vi "LED 2V2.vi"(0 "Digital IO in":T2, 5 "LED Red":bool, 9 "LED Green":bool, 11 "error in (no error)":errorcluster, 12 "LED Red 2":bool, 13 "LED Green 2":bool) -> (4 "Digital IO out":T1, 15 "error out":errorcluster)   [LabVIEW 2020]
uses:
  <vilib>/High Genius/HG_WSI_Tookit/Dependencies/Library/Digital Input and Output/Digital Input and Output.lvclass
  C:/Program Files (x86)/National Instruments/LabVIEW 2020/vi.lib/High Genius/HG_WSI_Tookit/Dependencies/Library/HG_LIB/HG_LIB.lvclass
  <vilib>/High Genius/HG_WSI_Tookit/Dependencies/Library/HG_LIB/HG_LIB.lvclass
  <vilib>/High Genius/HG_WSI_Tookit/Dependencies/Library/VMX Library.lvlib
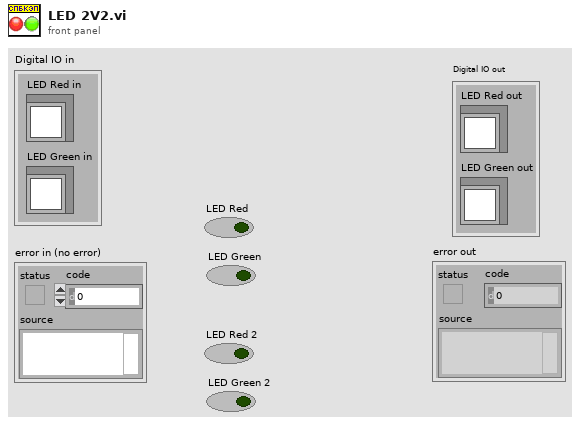
[diagram p1: front panel]
types:
  T1 = cluster{"LED Red out":refnum<class "Digital Input and Output.lvclass">, "LED Green out":refnum<class "Digital Input and Output.lvclass">}
  T2 = cluster{"LED Red in":refnum<class "Digital Input and Output.lvclass">, "LED Green in":refnum<class "Digital Input and Output.lvclass">}
  T3 = cluster{"Digital IO out":refnum<class "Digital Input and Output.lvclass">, "Digital IO out":refnum<class "Digital Input and Output.lvclass">}
  T4 = typedef "Semaphore RefNum" = refnum<k1>
  T5 = cluster{"titanenc0":i32, "titanenc1":i32, "titanenc2":i32, "titanenc3":i32, "rpm0":i16, "rpm1":i16, "rpm2":i16, "rpm3":i16, "resetenc0":bool, "resetenc1":bool, "resetenc2":bool, "resetenc3":bool}
  T6 = cluster{"data":cluster{"ai22":sgl, "ai23":sgl, "ai24":sgl, "ai25":sgl, "pulse12":i32, "pulse13":i32, "pwm14":i32, "pwm15":i32, "pwm16":dbl, "do17":bool, "do18":bool, "do19":bool, "do20":bool, "do21":bool, "di11":bool, "di9":bool, "motor0":u8, "motor1":u8, "motor2":u8, "motor3":u8, "dir00":u8, "dir01":u8, "dir02":u8, "dir03":u8, "dir10":u8, "dir11":u8, "dir12":u8, "dir13":u8, "limit0":bool, "limit1":bool, "limit2":bool, "limit3":bool, "limit4":bool, "limit5":bool, "limit6":bool, "limit7":bool, "lsb0H":u8, "lsb1H":u8, "lsb2H":u8, "lsb3H":u8, "lsb0L":u8, "lsb1L":u8, "lsb2L":u8, "lsb3L":u8, "enc0_counters":u32, "enc1_counters":u32, "enc2_counters":u32, "enc3_counters":u32, "counter10":u32, "counter8":u32, "reset_enc0":bool, "reset_enc1":bool, "reset_enc2":bool, "reset_enc3":bool, "pitch":sgl, "roll":sgl, "yaw":sgl, "zero_yaw":bool}}
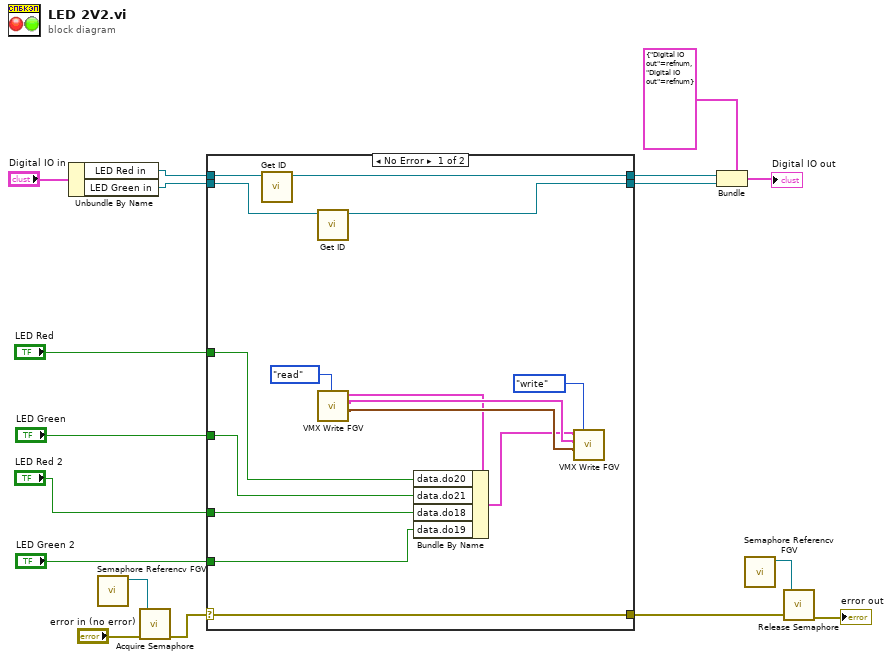
[diagram p0: block diagram]
diagram:
  n1 = Unbundle By Name("Digital IO in") -> ("LED Red in"=w4:refnum<class "Digital Input and Output.lvclass">, "LED Green in"=w3:refnum<class "Digital Input and Output.lvclass">)
  n2 = call <vilib>:"Semaphore Referencv FGV.vi"() -> ("Semaphore Reference"=w15:T4)  [unwired: 11 in]
  n3 = call <vilib>:"Acquire Semaphore.vi"("error in (no error)"="error in (no error)", "semaphore"=w15) -> ("error out"=w10:errorcluster)  [unwired: 3 in, 2 out]
  n4 = case shown="No Error" w10 {
    selector: w10 -> [w32 w35]
    tunnel: [w32 w35] -> w13
    tunnel: w4 -> [w31 w34]
    tunnel: [w30 w34] -> w9
    tunnel: w3 -> [w29 w33]
    tunnel: [w28 w33] -> w8
    tunnel: "LED Green" -> [w21 _]
    tunnel: "LED Red" -> [w20 _]
    tunnel: "LED Red 2" -> [w19 _]
    tunnel: "LED Green 2" -> [w18 _]
    frame No Error {
      n5 = call <vilib>:"Get ID.vi"("HG_LIB in"=w31) -> ("HG_LIB out"=w30:refnum<class "Digital Input and Output.lvclass">)  [unwired: 9 in, 1 out]
      n6 = call <vilib>:"Get ID.vi"("HG_LIB in"=w29) -> ("HG_LIB out"=w28:refnum<class "Digital Input and Output.lvclass">)  [unwired: 9 in, 1 out]
      n7 = call <vilib>:"VMX Write FGV.vi"("Enum"=enum16{"read", "write"}."read") -> ("Read Data3"=w25:cluster{"pwm17":i32, "pwm18":i32}, "Read Data2"=w26:T5, "Read Data"=w23:T6)  [unwired: 8 in]
      n8 = Bundle By Name(cluster=w23, "data.do20"=w20, "data.do21"=w21, "data.do18"=w19, "data.do19"=w18) -> (w22:T6)
      n9 = call <vilib>:"VMX Write FGV.vi"("Enum"=enum16{"read", "write"}."write", "Write Data3"=w25, "Write Data2"=w26, "Write Data"=w22) -> ()  [unwired: 5 in, 3 out]
    }
    frame Error {
    }
  }
  n10 = Bundle(cluster=T3 {"Digital IO out"=refnum, "Digital IO out"=refnum} ("Digital IO out"), "Digital IO out"=w9, "Digital IO out"=w8) -> (→"Digital IO out":T3)
  n11 = call <vilib>:"Semaphore Referencv FGV.vi"() -> ("Semaphore Reference"=w14:T4)  [unwired: 11 in]
  n12 = call <vilib>:"Release Semaphore.vi"("error in (no error)"=w13, "semaphore"=w14) -> ("error out"=→"error out":errorcluster)  [unwired: 4 in, 1 out]
